vi "Python@Script(Worker)__Parameter.vi"(1 "ParamterIn":string) -> (0 "ParamterOut":string)   [LabVIEW 2020]
panel:
  in  "Session":string(combo)
  in  "PythonCode":string
  in  "Confirm":bool
  # "Python@Script(Worker) Worker::$PythonCode"
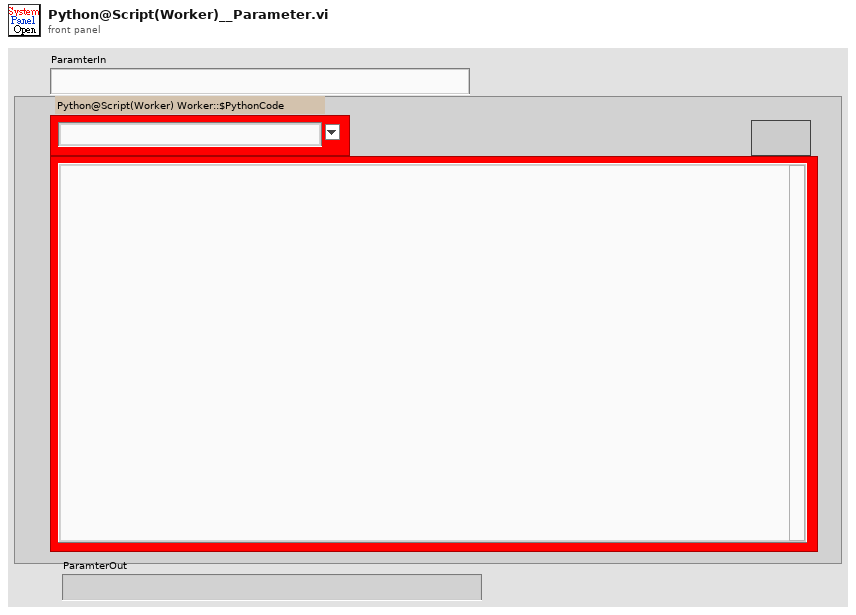
[diagram p1: front panel]
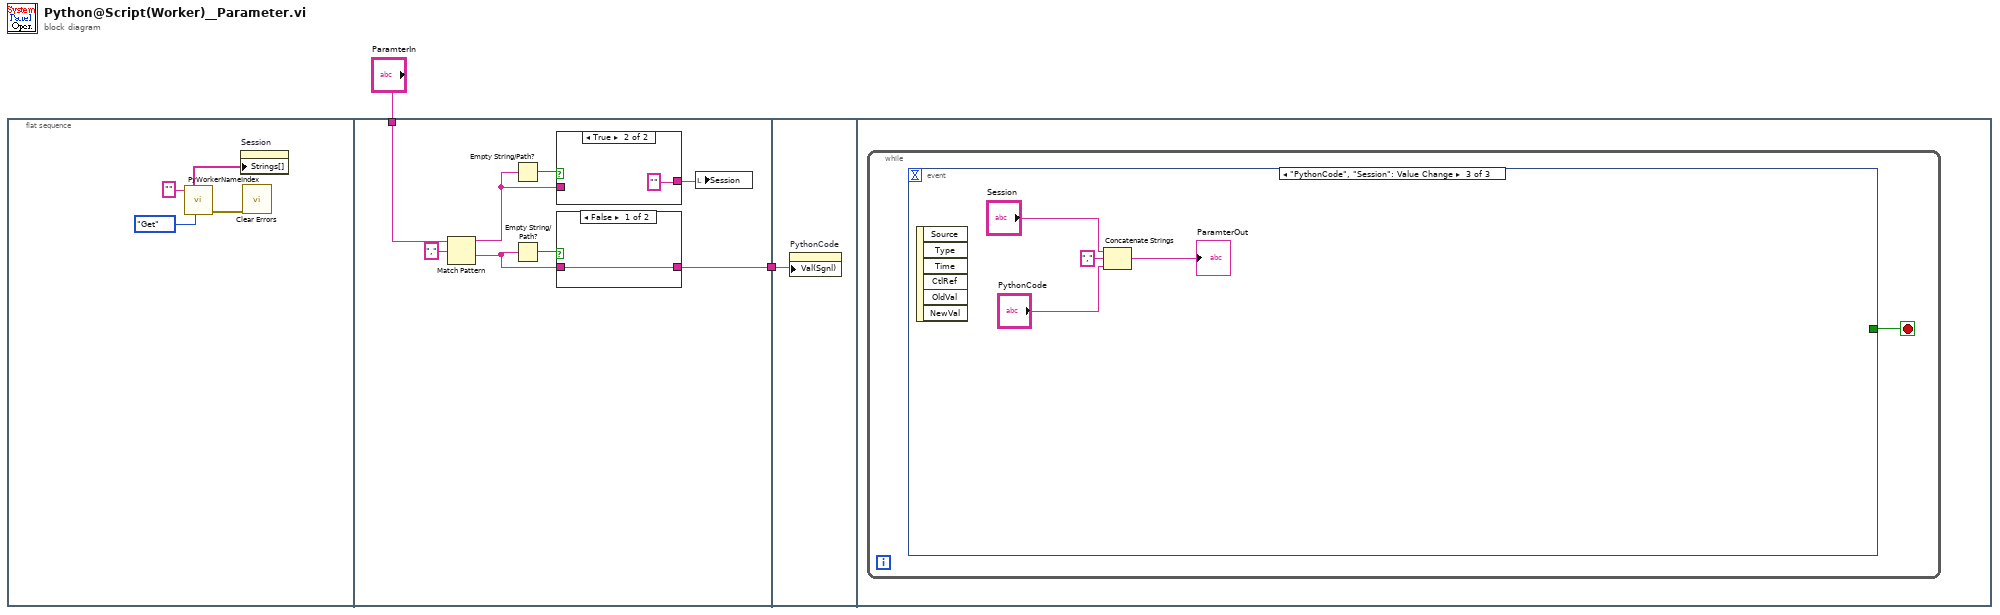
[diagram p0: block diagram]
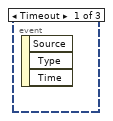
[diagram p4: hidden frame]
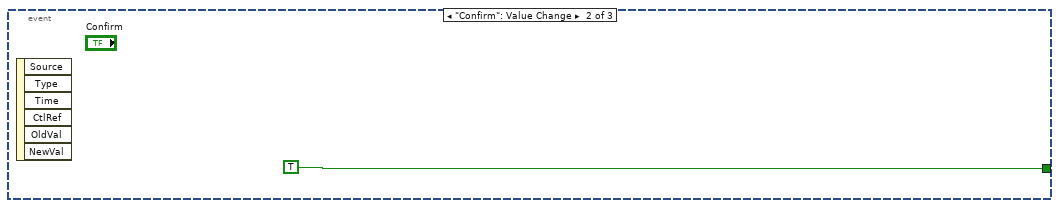
[diagram p5: hidden frame]
diagram:
  n1 = flat-sequence {
    tunnel: "ParamterIn" -> [w12]
    tunnel: [w13] -> w1
    tunnel: w1 -> [w19]
    frame #0 {
      n2 = call "PyWorkerNameIndex.vi"("OP"=enum16{"Init", "Get", "Set"}."Get", "WrokerName"="" ("SessionIn")) -> ("error out"=w3:errorcluster, "PythonWorkerNameS"=w5:string[])  [unwired: 6 in, 2 out]
      n3 = property on="Session" class="CmbBox"("Strings[]"=w5) -> ()  [unwired: 2 in, 2 out]
      n4 = call <vilib>:"Clear Errors.vi"("error in (no error)"=w3) -> ()  [unwired: 5 in, 2 out]
    }
    frame #1 {
      n5 = Match Pattern(string=w12, regular expression=",") -> (before substring=w8:string, after substring=w10:string)  [unwired: 1 in, 2 out]
      n6 = Empty String/Path?(string/path=w8) -> (empty?=w9:bool)
      n7 = Empty String/Path?(string/path=w10) -> (empty?=w14:bool)
      n8 = case shown="True" w9 {
        tunnel: w8 -> [w15 _]
        tunnel: [w15 ""] -> w7
        frame False {
        }
        frame True {
        }
      }
      n9 = case shown="False" w14 {
        tunnel: w10 -> [w17 w18]
        tunnel: [w17 w18] -> w13
        frame False {
        }
        frame True {
        }
      }
      n10 = local write "Session"(w7) -> ()
    }
    frame #2 {
      n11 = property on="PythonCode" class="Str"("Val(Sgnl)"=w19) -> ()  [unwired: 2 in, 2 out]
    }
    frame #3 {
      n12 = while {
        stop <- w20 stop-if-true
        n13 = event shown="[2] \"PythonCode\", \"Session\": Value Change" {
          selector: _ -> [_ _ _]
          dyn-events: _ -> [_ _ _]
          timeout: _ -> [_ _ _]
          tunnel: [_ TRUE _] -> w20
          event Timeout {
            n14 = event-data() -> ()  [unwired: 1 in, 3 out]
          }
          event "Confirm": Value Change {
            n15 = event-data() -> ()  [unwired: 1 in, 6 out]
          }
          event "PythonCode", "Session": Value Change {
            n16 = event-data() -> ()  [unwired: 1 in, 6 out]
            n17 = Concatenate Strings("Session", "," ("string"), "PythonCode") -> (→"ParamterOut":string)
          }
        }
      }
    }
  }
